vi "GenValveCalibrationSequence.vi"(9 "Ctr Odor Valve":u16(ring) items=["A1", "A2", "A3", "A4", "B1", "B2", "B3", "B4", "B5", "B6", "B7", "B8", "A5", "A6", "A7", "A8"], 10 "Water Mix Valve":u16(ring) items=["A1", "A2", "A3", "A4", "B1", "B2", "B3", "B4", "B5", "B6", "B7", "B8", "A5", "A6", "A7", "A8", ""], 11 "Valve List":u16[](array[numeric])) -> (3 "Valve Sequence Array":T1(array[cluster]))   [LabVIEW 2016]
panel:
  out "Array 2":u16[](array[numeric])
  in  "Flowboard":enum16{"A", "B", "C"}(ring)
  in  "Channel":enum16{"1", "2", "3", "4", "5", "6", "7", "8"}(ring)
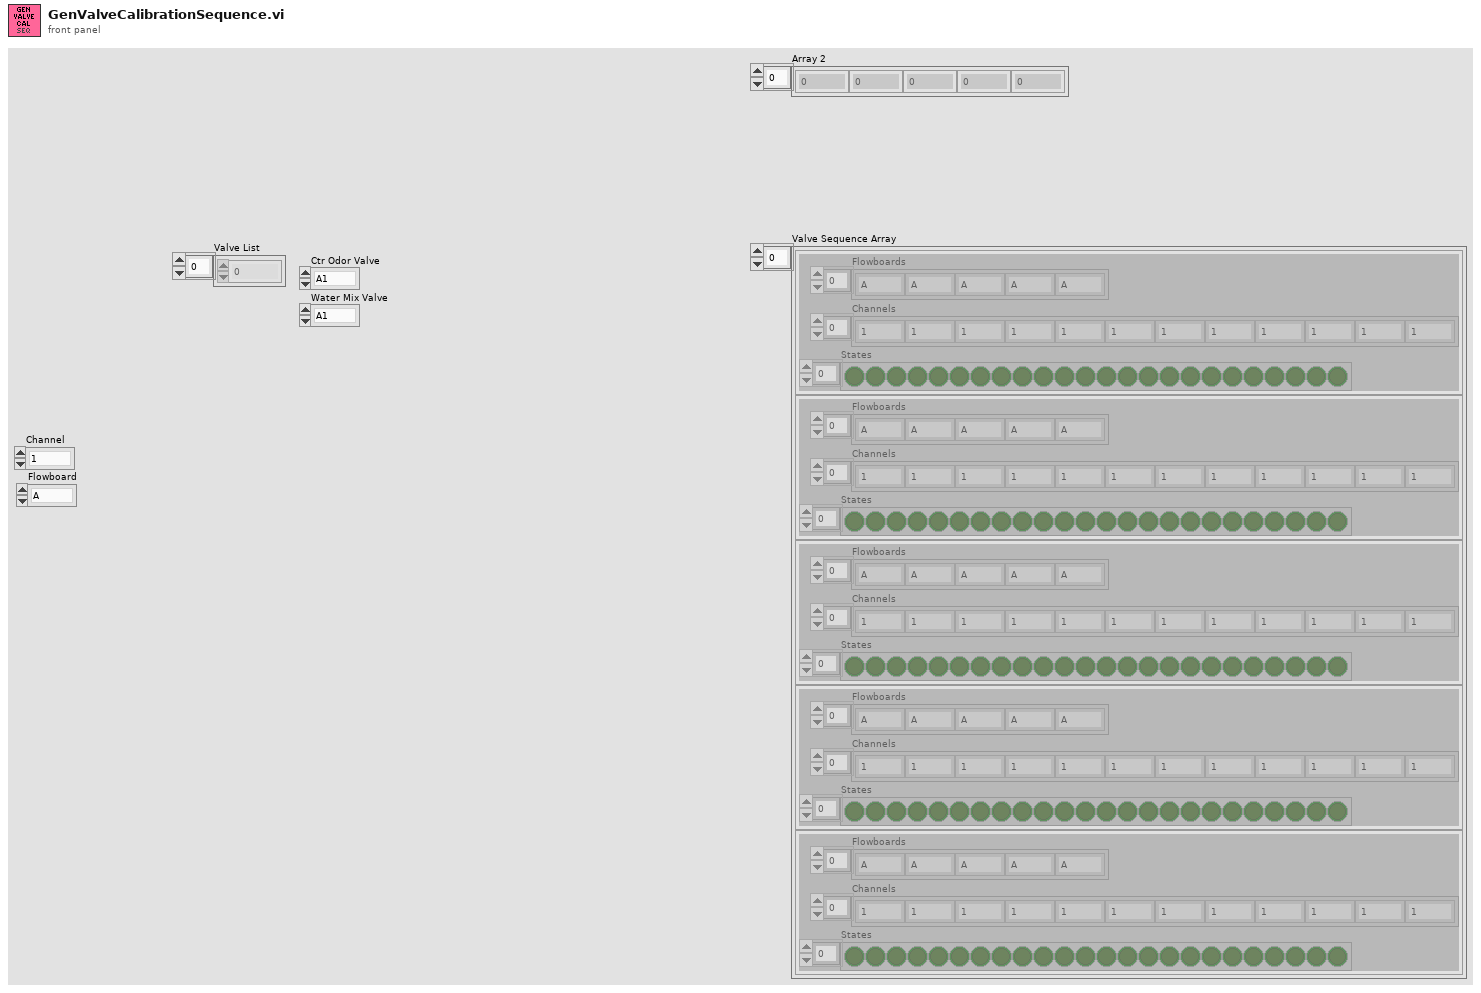
[diagram p1: front panel]
types:
  T1 = cluster{"Flowboards":enum16{"A", "B", "C"}[], "Channels":enum16{"1", "2", "3", "4", "5", "6", "7", "8"}[], "States":bool[]}[]
  T2 = cluster{"Flowboards":enum16{"A", "B", "C"}[], "Channels":enum16{"1", "2", "3", "4", "5", "6", "7", "8"}[], "States":bool[]}
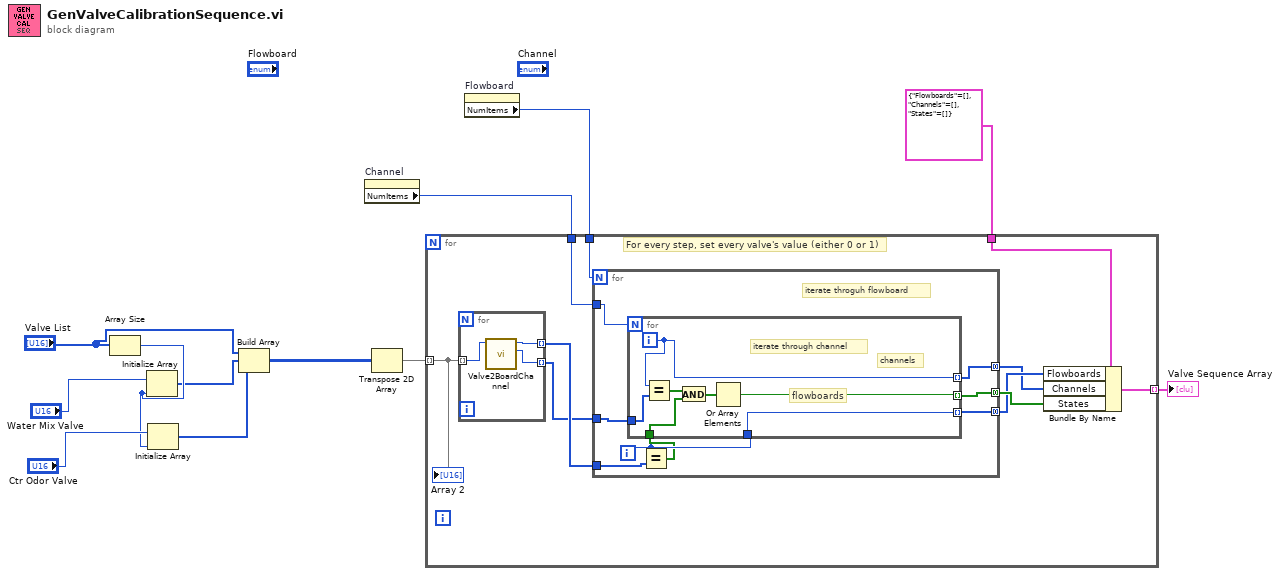
[diagram p0: block diagram]
diagram:
  n1 = Array Size(array="Valve List") -> (size(s)=w8:i32)
  n2 = Initialize Array("Water Mix Valve", w8) -> (w6:u16[])
  n3 = Initialize Array("Ctr Odor Valve", w8) -> (w5:u16[])
  n4 = Build Array("Valve List", w6, w5) -> (w4:u16[][])
  n5 = property on="Channel" class="Enum (strict)"() -> ("NumItems"=w1:u32)  [unwired: 2 in, 2 out]
  n6 = Transpose 2D Array(2D array=w4) -> (transposed array=w3:u16[][])
  n7 = property on="Flowboard" class="Enum (strict)"() -> ("NumItems"=w2:u32)  [unwired: 2 in, 2 out]
  n8 = for {
    tunnel: T2 {"Flowboards"=[], "Channels"=[], "States"=[]} ("Valve Data") -> [w22]
    tunnel: [w18] -> w11 mode=indexing
    tunnel: w2 -> [w15]
    tunnel: w1 -> [w14]
    tunnel: w3 -> [w13] mode=indexing
    # "For every step, set every valve's value (either 0 or 1)"
    n9 = for {
      tunnel: [w25] -> w17 mode=indexing
      tunnel: [w24] -> w16 mode=indexing
      tunnel: w13 -> [w23] mode=indexing
      n10 = call "Valve2BoardChannel.vi"("ValveID"=w23) -> ("Channel"=w24:enum16{"1", "2", "3", "4", "5", "6", "7", "8"}, "Flowboard"=w25:enum16{"A", "B", "C"})  [unwired: 9 in]
    }
    n11 = for {
      N: w15 -> [_]
      tunnel: w14 -> [w33]
      tunnel: [w32] -> w19 mode=concatenating
      tunnel: [w31] -> w20 mode=concatenating
      tunnel: w17 -> [w29]
      tunnel: w16 -> [w30]
      tunnel: [w26] -> w21 mode=concatenating
      i -> [w28]
      # "iterate throguh flowboard"
      n12 = Equal?(x=w28, y=w29) -> (x = y?=w27:bool[])
      n13 = for {
        N: w33 -> [_]
        tunnel: [w39] -> w32 mode=indexing
        tunnel: w28 -> [w38]
        tunnel: [w38] -> w31 mode=indexing
        tunnel: w30 -> [w40]
        tunnel: w27 -> [w36]
        tunnel: [w34] -> w26 mode=indexing
        i -> [w39]
        # "flowboards"
        # "channels"
        # "iterate through channel"
        n14 = Equal?(x=w39, y=w40) -> (x = y?=w37:bool[])
        n15 = And(x=w37, y=w36) -> (x .and. y?=w35:bool[])
        n16 = Or Array Elements(Boolean array=w35) -> (logical OR=w34:bool)
      }
    }
    n17 = Bundle By Name(cluster=w22, "Flowboards"=w20, "Channels"=w19, "States"=w21) -> (w18:T2)
    "Array 2" <- w13
  }
  "Valve Sequence Array" <- w11
